vi "draw.vi"(0 "reference":refnum<class "ImplicitParameterNode.lvclass">, 1 "graphics":refnum<class "Graphics.lvclass">, 5 "error in (no error)":errorcluster) -> (14 "reference out":refnum<class "ImplicitParameterNode.lvclass">, 19 "error out":errorcluster)   [LabVIEW 2020, in "ImplicitParameterNode.lvclass"]
doc: "public void draw(Graphics2D g2)"
uses:
  <resource>/Framework/Providers/Open_GDS/UML/ImplicitParameterNode_class/ImplicitParameterNode.lvclass
  C:/Program Files (x86)/National Instruments/LabVIEW 2020/resource/Framework/Providers/Open_GDS/UML/RectangularNode_class/RectangularNode.lvclass
  <resource>/Framework/Providers/Open_GDS/UML/Graphics_class/Graphics.lvclass
  <resource>/Framework/Providers/Open_GDS/UML/Graphics_class/StrokeType.ctl
  <resource>/Framework/Providers/Open_GDS/UML/General/Point/Point Point2D.ctl
  <resource>/Framework/Providers/Open_GDS/UML/MultiLineString_class/MultiLineString.lvclass
  <resource>/Framework/Providers/Open_GDS/UML/RectangularNode_class/RectangularNode.lvclass
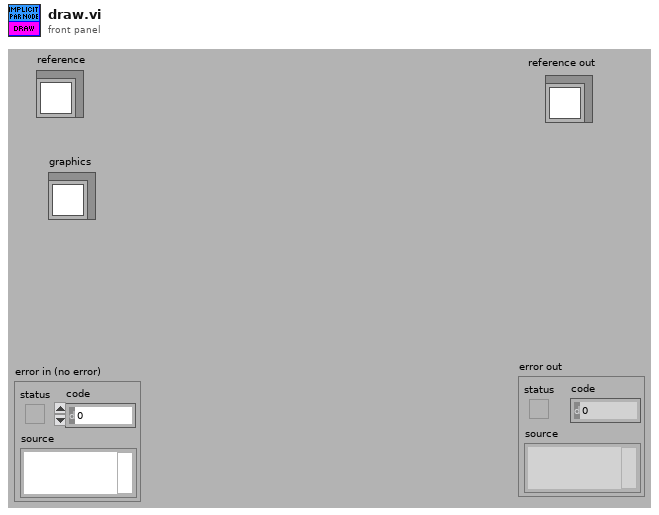
[diagram p1: front panel]
types:
  T1 = typedef "Graphics.lvclass/StrokeType.ctl" = enum16{"USE_DEFAULT", "SOLID", "DOTTED"}
  T2 = typedef "Point Point2D.ctl" = cluster{"x":dbl, "y":dbl}
  T3 = typedef "Rectangle Rectangle2D.ctl" = cluster{"x":dbl, "y":dbl, "width":dbl, "height":dbl}
  T4 = typedef "ImplicitParameterNode.lvclass/ObjectAttributes.ctl" = cluster{"topHeight":dbl, "name":refnum<class "MultiLineString.lvclass">, "DEFAULT_TOP_HEIGHT":i32, "DEFAULT_WIDTH":i32, "DEFAULT_HEIGHT":i32}
  T5 = typedef "RectangularNode.lvclass/ObjectAttributes.ctl" = cluster{"bounds":T3}
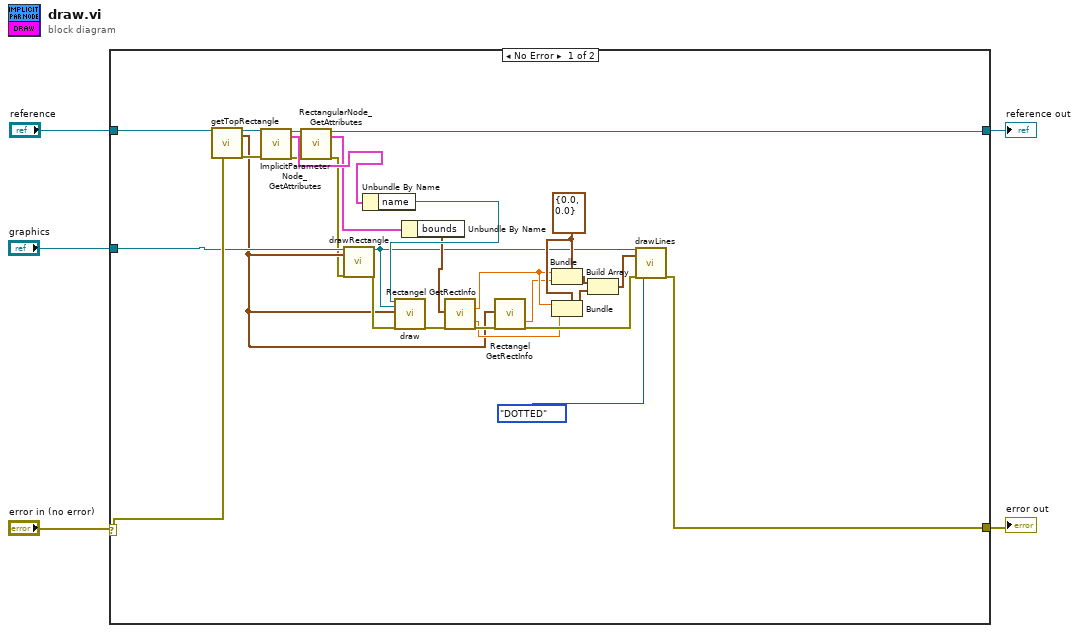
[diagram p0: block diagram]
diagram:
  n1 = case shown="No Error" "error in (no error)" {
    selector: "error in (no error)" -> [w31 w34]
    tunnel: "reference" -> [w33 w35]
    tunnel: [w32 w34] -> w4
    tunnel: [w7 w35] -> w3
    tunnel: "graphics" -> [w30 _]
    frame No Error {
      w20 = T2 {"x"=0.0, "y"=0.0} ("point2D")
      n2 = call-dynamic "getTopRectangle.vi"("reference"=w33, "error in (no error)"=w31) -> ("reference out"=w28:refnum<class "ImplicitParameterNode.lvclass">, "bounds"=w12:T3, "error out"=w27:errorcluster)  [unwired: 15 in]
      n3 = call <resource>:"ImplicitParameterNode_GetAttributes.vi"("reference in"=w28, "error in (no error)"=w27) -> ("reference out"=w10:refnum<class "ImplicitParameterNode.lvclass">, "Data"=w11:T4, "error out"=w9:errorcluster)  [unwired: 1 in, 14 out]
      n4 = call <resource>:"RectangularNode_GetAttributes.vi"("reference in"=w10, "error in (no error)"=w9) -> ("reference out"=w7:refnum<class "ImplicitParameterNode.lvclass">, "Data"=w6:T5, "error out"=w8:errorcluster)  [unwired: 14 in, 1 out]
      n5 = call <resource>:"drawRectangle.vi"("reference"=w30, "rectangle"=w12, "error in (no error)"=w8) -> ("reference out"=w13:refnum<class "Graphics.lvclass">, "error out"=w29:errorcluster)  [unwired: 4 in, 11 out]
      n6 = Unbundle By Name(w11) -> ("name"=w26:refnum<class "MultiLineString.lvclass">)
      n7 = call-dynamic "draw.vi"("reference"=w26, "graphics"=w13, "bounds"=w12, "error in (no error)"=w29) -> ("error out"=w25:errorcluster)  [unwired: 14 in, 1 out]
      n8 = Unbundle By Name(w6) -> ("bounds"=w24:T3)
      n9 = call <resource>:"Rectangel GetRectInfo.vi"("bounds"=w24, "error in (no error)"=w25) -> ("centerX"=w16:dbl, "maxY"=w14:dbl, "error out"=w23:errorcluster)  [unwired: 15 out]
      n10 = call <resource>:"Rectangel GetRectInfo.vi"("bounds"=w12, "error in (no error)"=w23) -> ("maxY"=w15:dbl, "error out"=w21:errorcluster)  [unwired: 16 out]
      n11 = Bundle(cluster=w20, "x"=w16, "y"=w15) -> (w19:T2)
      n12 = Bundle(cluster=w20, "x"=w16, "y"=w14) -> (w18:T2)
      n13 = Build Array(w19, w18) -> (w17:T2[])
      n14 = call <resource>:"drawLines.vi"("reference"=w13, "points"=w17, "error in (no error)"=w21, "stroke"=StrokeType."DOTTED") -> ("error out"=w32:errorcluster)  [unwired: 3 in, 12 out]
    }
    frame Error {
    }
  }
  "reference out" <- w3
  "error out" <- w4
